vi "PH_Beckhoff-16BB_Testtool.constructor.vi"(0 "name":string, 2 "data in":string, 5 "error in(no error)":errorcluster) -> (14 "i ref out":refnum<vi>, 16 "data out":string, 19 "error out":errorcluster)   [LabVIEW 2014, in "PH_Beckhoff-16BB_Testtool.lvlib"]
doc: "This class is forseen to control black boxes (motion).\n\nThis class is part of the PHELIX device layer.\n\nauthor: Stefan Götte, GSI\n\nLicense Agreement for this software:\n\nCopyright (C)\nGesellschaft für Schwerionenforschung, GSI\nPlanckstr. 1\n64291 Darmstadt\nGermany\n\nContact: D.Beck@gsi.de \n\nThis program is free software; you can redistribute it and/or modify it under the terms of the \nGNU General Public License as published by the Free Software Foundation; either version 2 of \nthe license, or (at your option) any later version.\n\nThis program is distributed in the hope that it will be useful, but WITHOUT ANY WARRANTY; \nwithout even the implied warranty of MERCHANTABILITY or FITNESS FOR A PARTICULAR PURPOSE. See the GNU General License for more details (http://www.gnu.org).\n\nGesellschaft für Schwerionenforschung, GSI\nPlanckstr. 1, 64291 Darmstadt, Germany\nFor all questions and ideas contact: M.Richter@gsi.de, H.Brand@gsi.de or D.Beck@gsi.de.\nLast update: 16-JUN-2004"
uses:
  PH_Beckhoff-16BB_Testtool.lvlib
  PH_Beckhoff-16BB_Testtool.i attribute.ctl
  CS_Core/CSObj/CSObj.lvlib
  PH_Basics/PH_Class/PH_Class.lvlib
  PH_Basics/PH_Common/PH_Common.lvlib
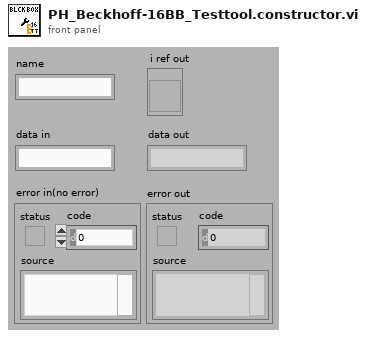
[diagram p1: front panel]
types:
  T1 = typedef "PH_Beckhoff-16BB_Testtool.lvlib/PH_Beckhoff-16BB_Testtool.i attribute.ctl" = cluster{"GUI Refs":refnum<vi>[], "16BB Instance":string}
  T2 = enum16{"SetAttribute", "GetAttribute", "CreateAttribute", "DestroyAttribute", "DestroyAllAtributes"}
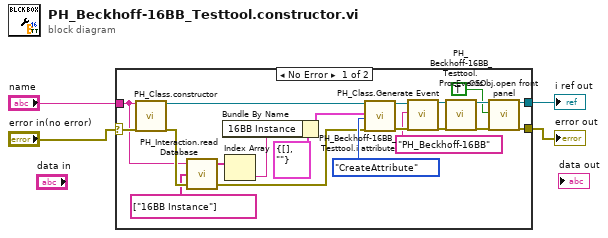
[diagram p0: block diagram]
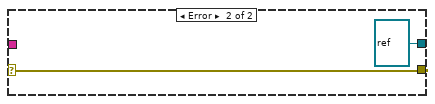
[diagram p2: hidden frame]
diagram:
  n1 = case shown="No Error" "error in(no error)" {
    selector: "error in(no error)" -> [w22 w27]
    tunnel: [w16 refnum<vi> refnum ("i ref out")] -> w4
    tunnel: [w18 w27] -> w3
    tunnel: "name" -> [w7 _]
    frame No Error {
      n2 = call "PH_Class.constructor.vi"("name"=w7, "error in"=w22) -> ("i ref out"=w23:refnum<vi>, "error out"=w24:errorcluster)  [unwired: 15 in, 1 out]
      n3 = call "PH_Interaction.read Database.vi"("error in (no error)"=w24, "Strings to search for"=string[] ["16BB Instance"], "DB Entry to read"=w7) -> ("error out"=w11:errorcluster, "Values"=w10:string[])  [unwired: 1 in]
      n4 = Index Array(array=w10) -> (element=w8:string)  [unwired: 1 in]
      n5 = Bundle By Name(cluster=T1 {"GUI Refs"=[], "16BB Instance"=""} ("CLASS.i attribute"), "16BB Instance"=w8) -> (w9:T1)
      n6 = call "PH_Beckhoff-16BB_Testtool.i attribute.vi"("VI Refnum"=w23, "CLASS.i attribute"=w9, "Action"=T2."CreateAttribute", "error in (no error)"=w11) -> ("VI Refnum out"=w13:refnum<vi>, "error out"=w14:errorcluster)  [unwired: 13 in, 1 out]
      n7 = call "PH_Class.Generate Event.vi"("i ref in"=w13, "Class"="PH_Beckhoff-16BB", "error in (no error)"=w14) -> ("i ref out"=w21:refnum<vi>, "error out"=w20:errorcluster)  [unwired: 15 in]
      n8 = call "PH_Beckhoff-16BB_Testtool.ProcEvents.vi"("i ref in"=w21, "error in (no error)"=w20) -> ("i ref out"=w17:refnum<vi>, "error out"=w19:errorcluster)  [unwired: 16 in]
      n9 = call "CSObj.open front panel.vi"("i ref in"=w17, "frontPanelOpen"=TRUE, "error in (no error)"=w19) -> ("i ref out"=w16:refnum<vi>, "error out"=w18:errorcluster)  [unwired: 15 in]
    }
    frame Error {
    }
  }
  "i ref out" <- w4
  "error out" <- w3
